vi "Door Open Interlock Value Change.vi"(8 "error in (no error)":errorcluster, 10 "Door Open Interlock":bool, 11 "Door Controller API in":refnum<class "Door Controller API.lvclass">) -> (0 "error out":errorcluster, 3 "Door Controller API out":refnum<class "Door Controller API.lvclass">)   [LabVIEW 2020, in "Door Controller API.lvlib" / "Door Controller API.lvclass"]
uses:
  Door Controller API.lvclass
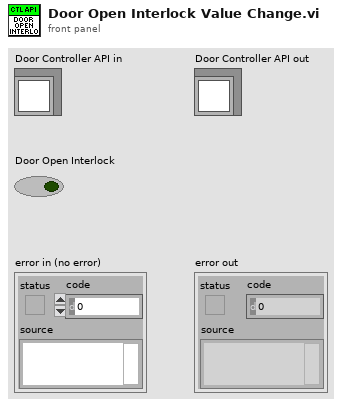
[diagram p1: front panel]
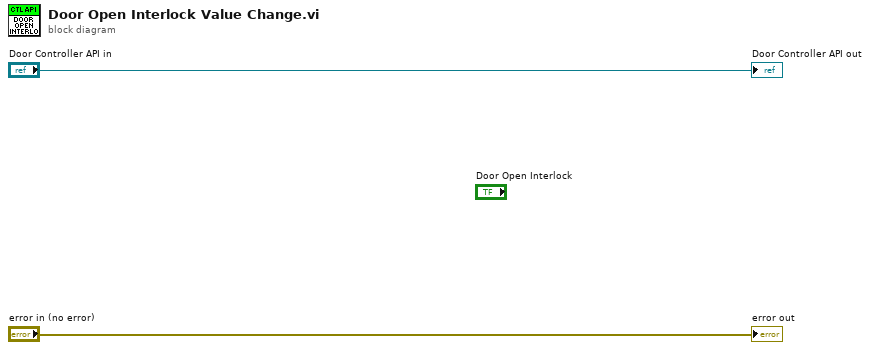
[diagram p0: block diagram]
diagram:
  "error out" <- "error in (no error)"
  "Door Controller API out" <- "Door Controller API in"
